vi "C.vi"(3 "t":ext, 4 "n^2":ext, 5 "Promien krzywizny południka [v]":ext, 6 "fi[rad]":ext) -> (0 "C":ext)   [LabVIEW 2012, in "Biblioteka moduł map v3.lvlib" / "Konwersja wsp.lvlib" / "UTM.lvlib" / "Konwersja na UTM.lvlib"]
doc: "Współczynnik wzoru na konwersję na UTM."
uses:
  Konwersja na UTM.lvlib
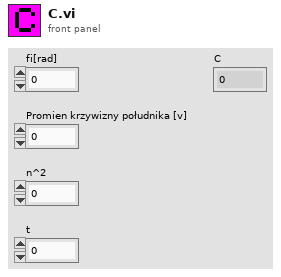
[diagram p1: front panel]
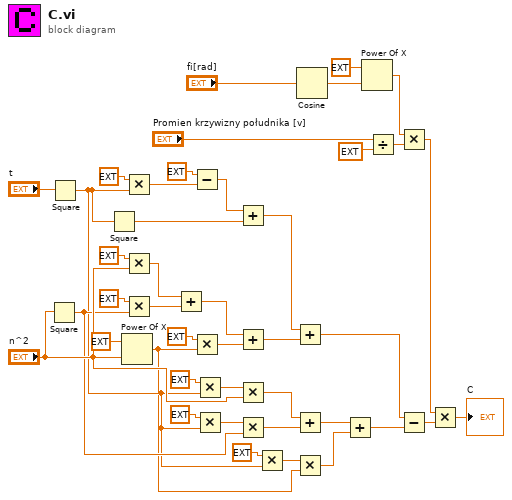
[diagram p0: block diagram]
diagram:
  n1 = Square(x="n^2") -> (x^2=w10:ext)
  n2 = Square(x="t") -> (x^2=w5:ext)
  n3 = Square(x=w5) -> (x^2=w28:ext)
  n4 = Power Of X(1:"n^2", 2:ext 3.0 ("y")) -> (0:w4:ext)
  n5 = Multiply(x=ext 18.0, y=w5) -> (x*y=w30:ext)
  n6 = Multiply(x=ext 14.0, y="n^2") -> (x*y=w26:ext)
  n7 = Multiply(x=ext 13.0, y=w10) -> (x*y=w24:ext)
  n8 = Add(x=w26, y=w24) -> (x+y=w23:ext)
  n9 = Subtract(x=ext 5.0, y=w30) -> (x-y=w29:ext)
  n10 = Multiply(x=ext 4.0, y=w4) -> (x*y=w21:ext)
  n11 = Multiply(x=ext 58.0, y=w5) -> (x*y=w15:ext)
  n12 = Multiply(x=ext 64.0, y=w5) -> (x*y=w11:ext)
  n13 = Add(x=w29, y=w28) -> (x+y=w19:ext)
  n14 = Add(x=w23, y=w21) -> (x+y=w18:ext)
  n15 = Multiply(x=w15, y="n^2") -> (x*y=w13:ext)
  n16 = Multiply(x=w11, y=w10) -> (x*y=w9:ext)
  n17 = Multiply(x=ext 24.0, y=w5) -> (x*y=w8:ext)
  n18 = Add(x=w19, y=w18) -> (x+y=w17:ext)
  n19 = Add(x=w13, y=w9) -> (x+y=w3:ext)
  n20 = Multiply(x=w8, y=w4) -> (x*y=w6:ext)
  n21 = Cosine(x="fi[rad]") -> (cos(x)=w37:ext)
  n22 = Add(x=w3, y=w6) -> (x+y=w2:ext)
  n23 = Power Of X(1:w37, 2:ext 5.0 ("y")) -> (0:w39:ext)
  n24 = Divide(x="Promien krzywizny południka [v]", y=ext 120.0) -> (x/y=w40:ext)
  n25 = Multiply(x=w39, y=w40) -> (x*y=w41:ext)
  n26 = Subtract(x=w17, y=w2) -> (x-y=w1:ext)
  n27 = Multiply(x=w41, y=w1) -> (x*y=→"C":ext)
